vi "STOP_ALL.vi"(10 "argv":string[](array[string]), 11 "args":u8) -> ()   [LabVIEW 2014]
uses:
  Robot Global Data.vi
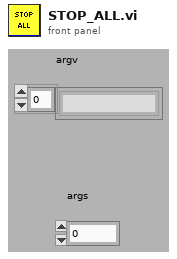
[diagram p1: front panel]
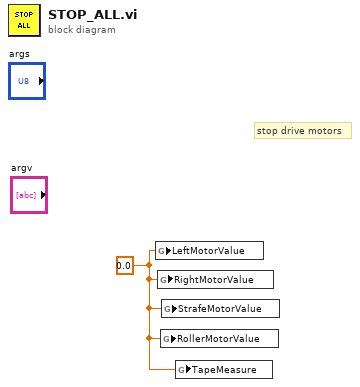
[diagram p0: block diagram]
diagram:
  w1 = 0.0 ("RightMotorValue")
  # "stop drive motors"
  n1 = global write "Robot Global Data.vi" "LeftMotorValue"(w1) -> ()
  n2 = global write "Robot Global Data.vi" "RightMotorValue"(w1) -> ()
  n3 = global write "Robot Global Data.vi" "RollerMotorValue"(w1) -> ()
  n4 = global write "Robot Global Data.vi" "StrafeMotorValue"(w1) -> ()
  n5 = global write "Robot Global Data.vi" "TapeMeasure"(w1) -> ()
